vi "Apply DM command and take picture.vi"(0 "Error in":errorcluster, 7 "WavefrontCorrector in":refnum<class "WavefrontCorrector.lvclass">, 8 "Offset positions":sgl[](graph), 9 "trigger time (ms)":dbl format="%#_13g", 10 "# of pictures":i32=1, 11 "path and file name, no .tif at the end":string="_groundtruth_") -> (6 "Error out":errorcluster)   [LabVIEW 2018]
uses:
  <userlib>/WaveKit.lib/Classes/WavefrontCorrector/WavefrontCorrector.lvclass
panel:
  in  "EMCCD trigger port":tag="Dev1/port0/line0"
  # "CANNOT run independently, casao nor EMCCD not initialized in this program"
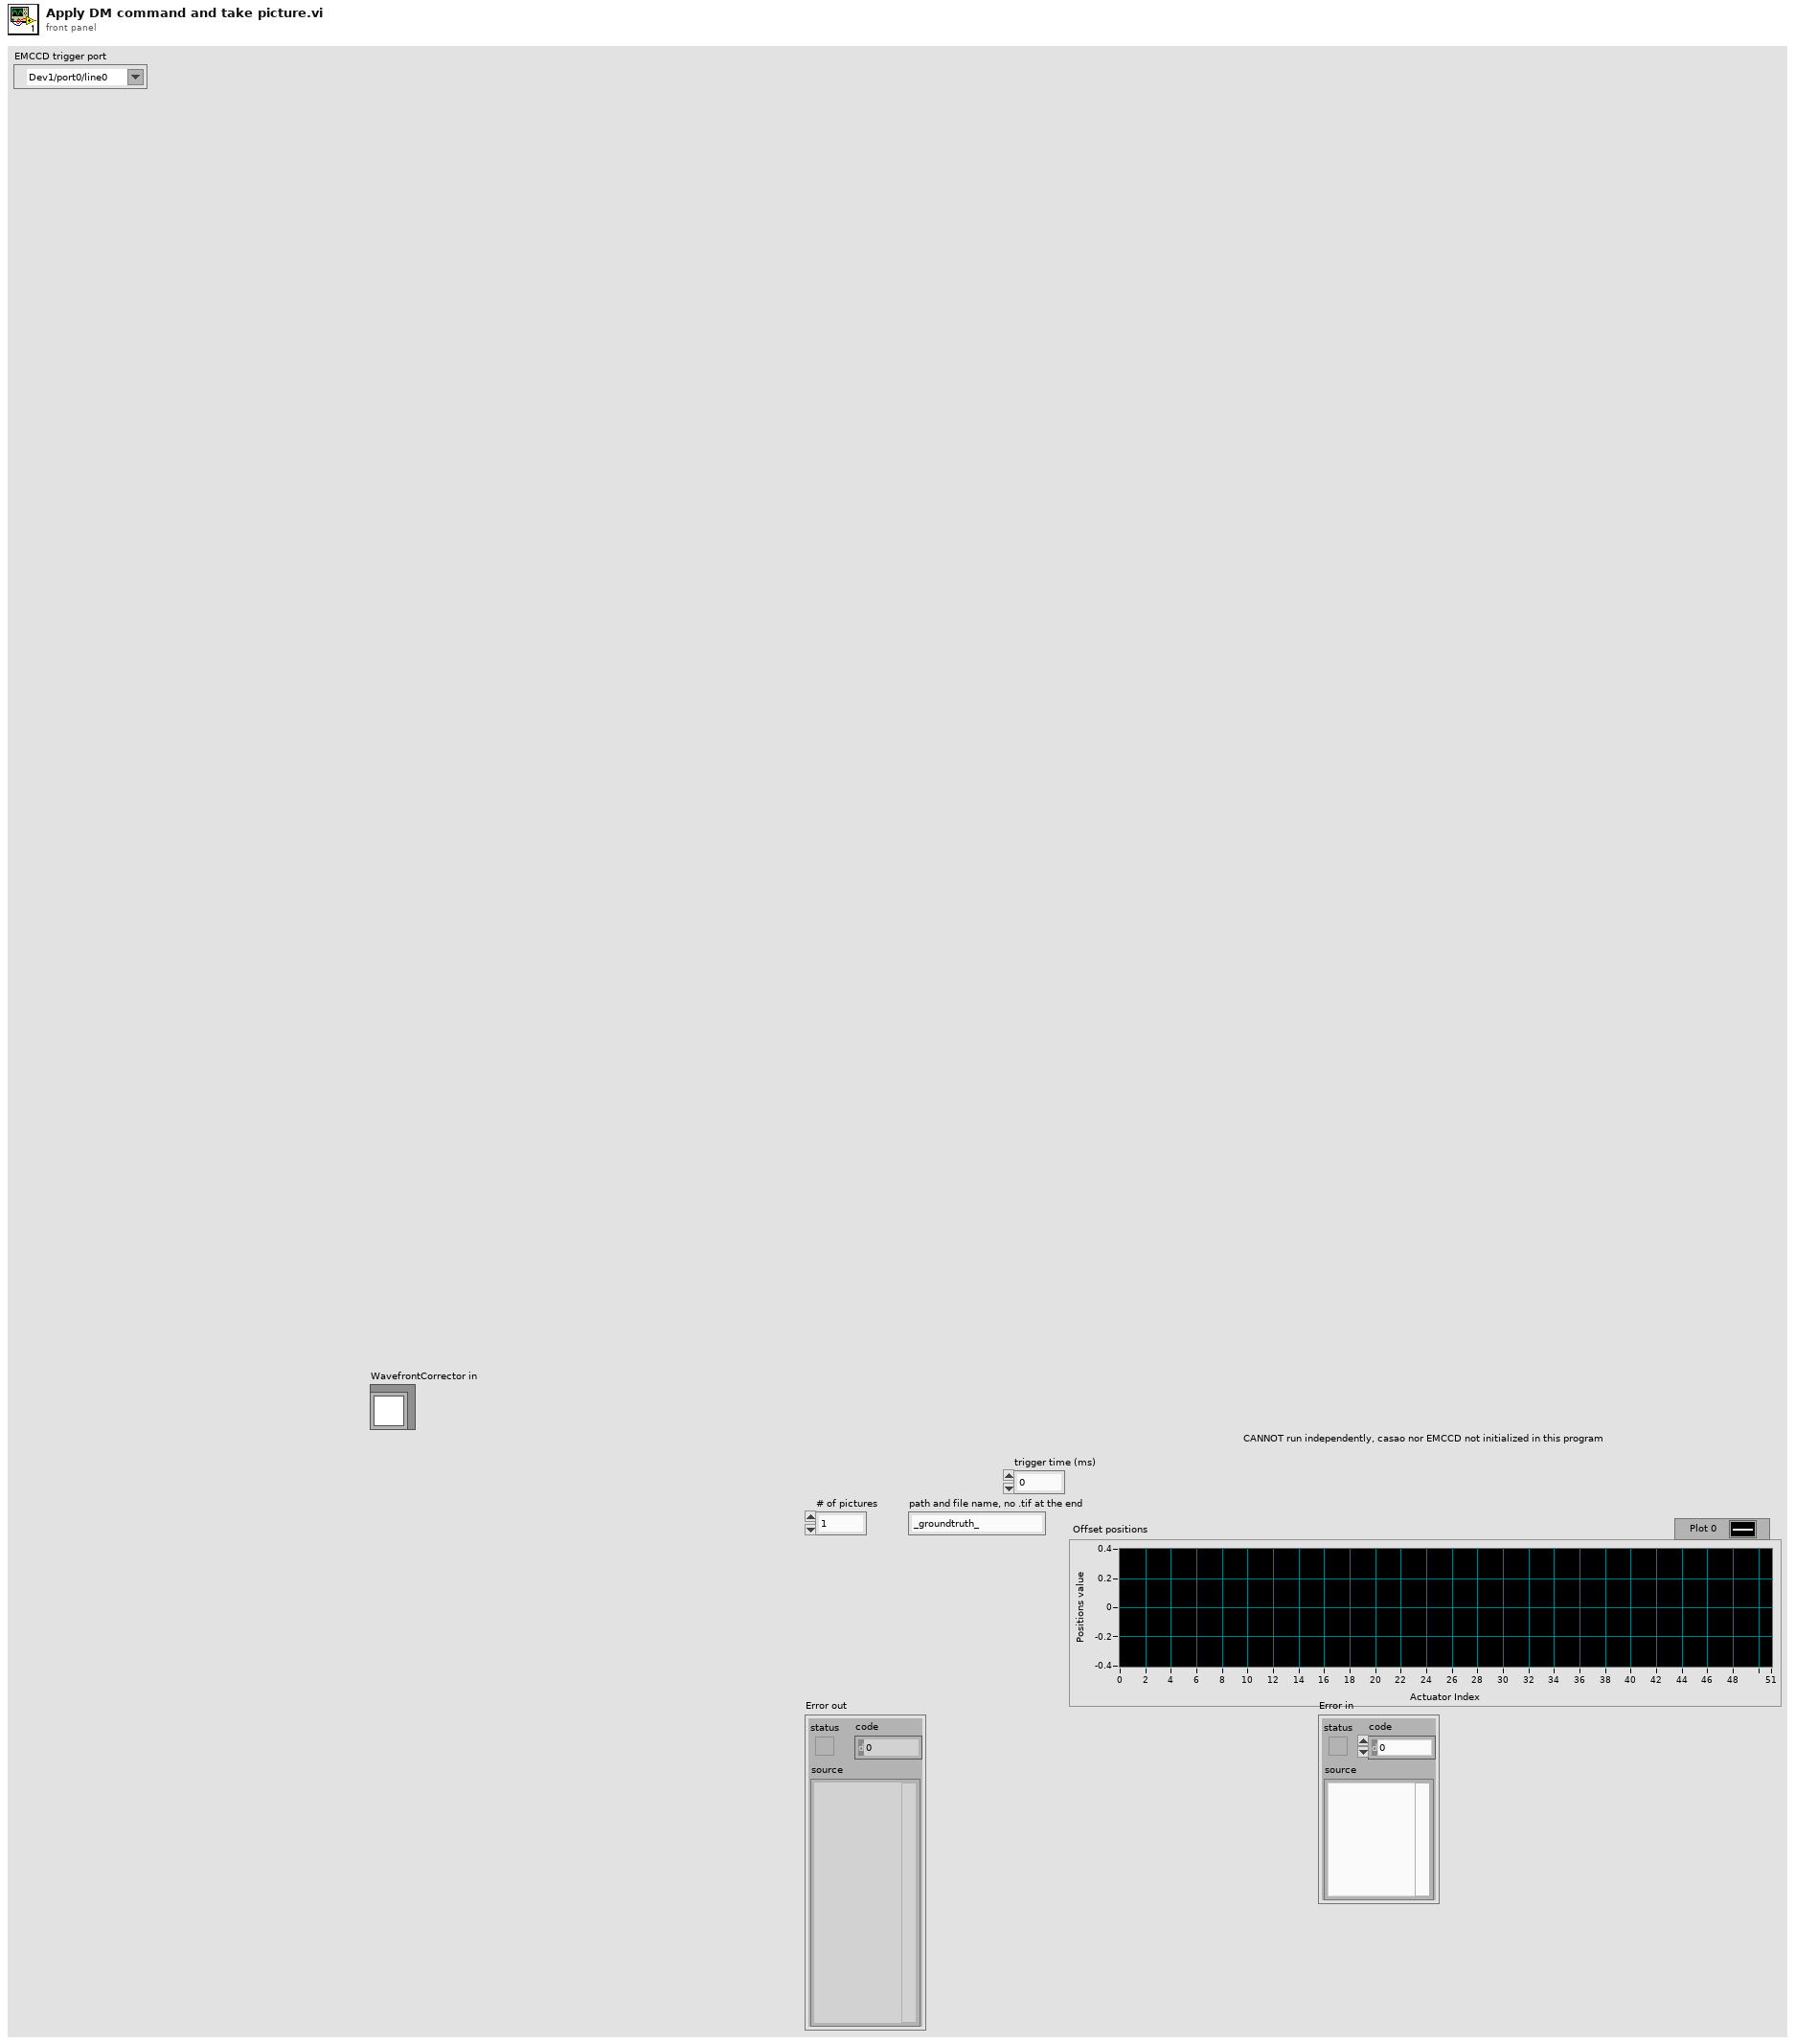
[diagram p1: front panel]
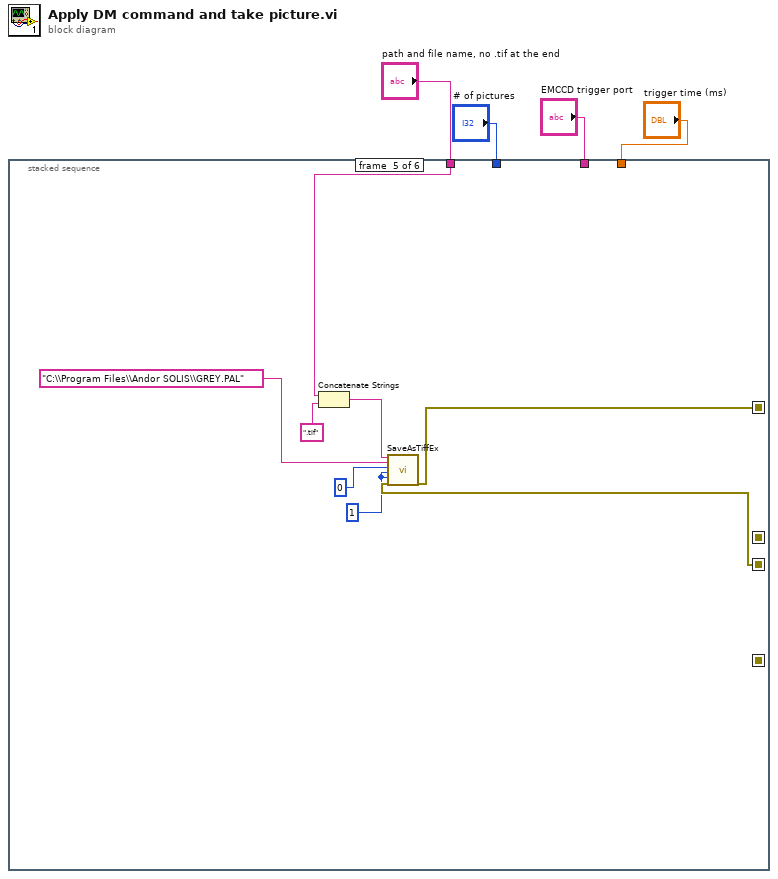
[diagram p0: block diagram]
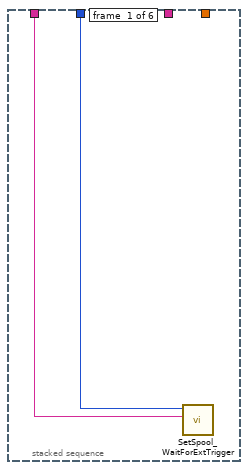
[diagram p2: hidden frame]
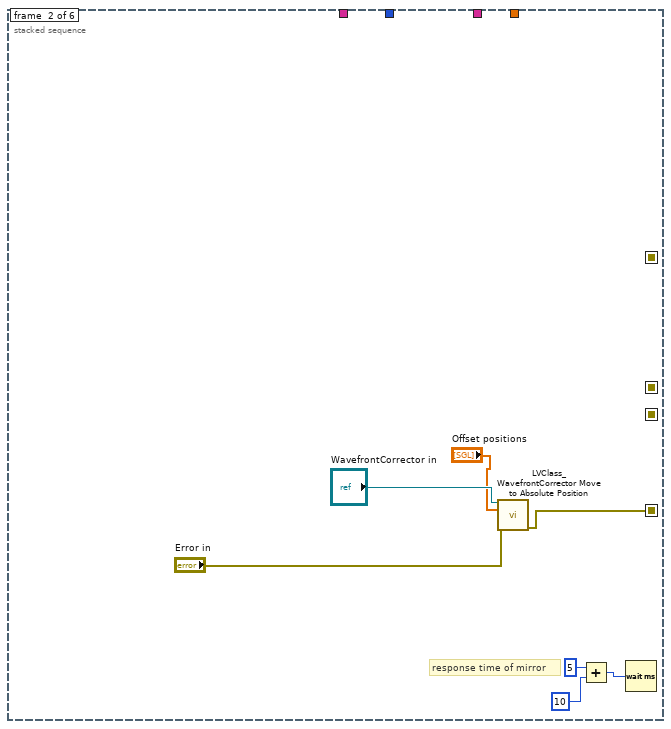
[diagram p3: hidden frame]
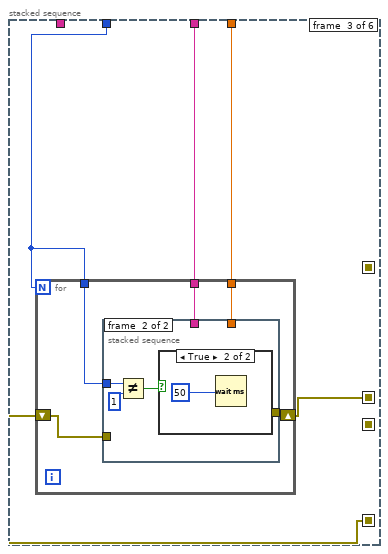
[diagram p4: hidden frame]
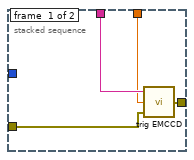
[diagram p5: hidden frame]
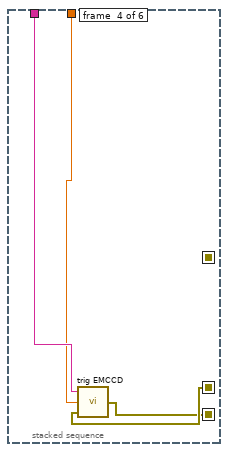
[diagram p7: hidden frame]
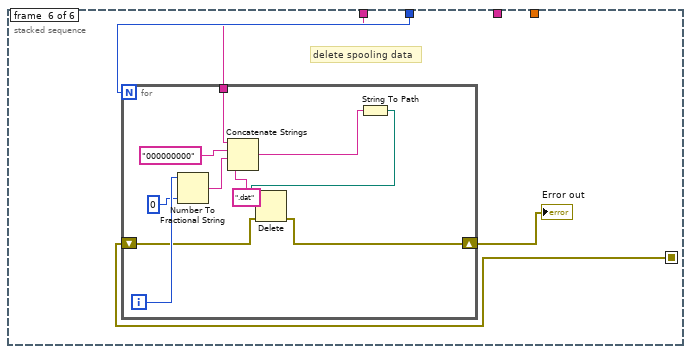
[diagram p8: hidden frame]
diagram:
  n1 = stacked-sequence {
    seq-local: [_ w7 _ _ _ _] -> [_ _ w16 _ _ _]
    seq-local: [_ _ w15 _ _ _] -> [_ _ _ w33 _ _]
    seq-local: [_ _ _ w32 _ _] -> [_ _ _ _ w38 _]
    seq-local: [_ _ _ _ w37 _] -> [_ _ _ _ _ w45]
    tunnel: "# of pictures" -> [w6 _ w14 _ _ w47]
    tunnel: "EMCCD trigger port" -> [_ _ w18 w35 _ _]
    tunnel: "trigger time (ms)" -> [_ _ w17 w34 _ _]
    tunnel: "path and file name, no .tif at the end" -> [w5 _ _ _ w40 w46]
    frame #0 {
      n2 = call "SetSpool_WaitForExtTrigger.vi"("path and name"=w5, "Kinetic Series"=w6) -> ()  [unwired: 10 in]
    }
    frame #1 {
      # "response time of mirror"
      n3 = call <userlib>:"LVClass_WavefrontCorrector Move to Absolute Position.vi"("WavefrontCorrector in"="WavefrontCorrector in", "Absolute Positions"="Offset positions", "error in (no error)"="Error in") -> ("error out"=w7:errorcluster)  [unwired: 11 in, 1 out]
      n4 = Add(x=5, y=10) -> (x+y=w11:i32)
      n5 = Wait (ms)(milliseconds to wait=w11) -> ()  [unwired: 1 out]
    }
    frame #2 {
      n6 = for {
        N: w14 -> [_]
        tunnel: w18 -> [w23]
        tunnel: w17 -> [w22]
        shift-right: [w21] -> w15
        shift-left: w16 -> [w20]
        tunnel: w14 -> [w19]
        n7 = stacked-sequence {
          tunnel: w23 -> [w27 _]
          tunnel: w22 -> [w26 _]
          tunnel: [w25 _] -> w21
          tunnel: w20 -> [w24 _]
          tunnel: w19 -> [_ w28]
          frame #0 {
            n8 = call "trig EMCCD.vi"("error in (no error)"=w24, "exp time (ms)"=w26, "lines"=w27) -> ("error out"=w25:errorcluster)
          }
          frame #1 {
            n9 = Not Equal?(x=w28, y=1) -> (x != y?=w30:bool)
            n10 = case shown="True" w30 {
              frame False {
              }
              frame True {
                n11 = Wait (ms)(milliseconds to wait=50) -> ()  [unwired: 1 out]
              }
            }
          }
        }
      }
    }
    frame #3 {
      n12 = call "trig EMCCD.vi"("error in (no error)"=w33, "exp time (ms)"=w34, "lines"=w35) -> ("error out"=w32:errorcluster)
    }
    frame #4 {
      w36 = 1
      n13 = Concatenate Strings(w40, ".tif") -> (w39:string)
      n14 = call <userlib>:"SaveAsTiffEx.vi"("path"=w39, "palette"="C:\\Program Files\\Andor SOLIS\\GREY.PAL", "position"=0, "type"=w36, "mode"=w36, "error in (no error)"=w38) -> ("error out"=w37:errorcluster)  [unwired: 12 in, 1 out]
    }
    frame #5 {
      # "delete spooling data"
      n15 = for {
        N: w47 -> [_]
        tunnel: w46 -> [w50]
        shift-right: [w48] -> w44
        shift-left: w45 -> [w49]
        i -> [w55]
        n16 = Number To Fractional String(number=w55, precision (6)=0) -> (F-format string=w53:string)  [unwired: 2 in]
        n17 = Concatenate Strings(w50, "000000000", w53, ".dat") -> (w52:string)
        n18 = String To Path(string=w52) -> (path=w57:path)
        n19 = Delete(path (use dialog)=w57, error in=w49) -> (error out=w48:errorcluster)  [unwired: 3 in, 2 out]
      }
      "Error out" <- w44
    }
  }
